vi "Untitled 2.vi"() -> ()   [LabVIEW 2016]
panel:
  out "String":string
  in  "Numeric":dbl
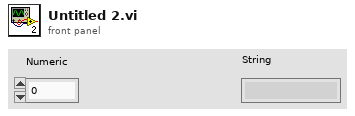
[diagram p1: front panel]
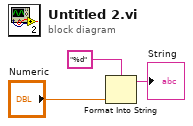
[diagram p0: block diagram]
diagram:
  n1 = Format Into String(format string="%d", "Numeric") -> (resulting string=→"String":string)  [unwired: 2 in, 1 out]
